vi "Runtime Test.vi"() -> ()   [LabVIEW 2017, in "WaveformAcq tests.lvlib"]
uses:
  WaveformAcq tests.lvlib
  <vilib>/NI/Tag Bus Module Framework/channel/channel classification.ctl
  <vilib>/NI/Tag Bus/tag/Data Type.ctl
  module/configuration/WaveformAcq configuration.lvclass
  C:/Program Files (x86)/National Instruments/LabVIEW 2017/vi.lib/NI/Configuration Framework/serializable configuration/NISE_CEF_serializable configuration.lvclass
  C:/Program Files (x86)/National Instruments/LabVIEW 2017/vi.lib/NI/Tag Bus Module Framework/module configuration/TBM module configuration.lvclass
  module/execution/WaveformAcq runtime.lvclass
  <vilib>/NI/Tag Bus/dictionary/data dictionary.lvclass/data dictionary.ctl
  <vilib>/NI/Tag Bus/dictionary/lookup polymorphs/locate double.vi
  <vilib>/NI/Tag Bus/table/data polymorphs/write one/write Double.vi
  <vilib>/NI/Tag Bus/table/data polymorphs/read one/read Double.vi
  <vilib>/NI/Tag Bus/dictionary/search/find data index.vi
  <vilib>/NI/Tag Bus/dictionary/search/search string list.vi
  <vilib>/NI/Tag Bus/dictionary/tag not found.vi
  <vilib>/NI/Tag Bus Module Framework/channel/TBM channel.lvclass
  <vilib>/NI/Tag Bus/tag/tag descriptor.lvclass
  <vilib>/NI/Tag Bus/dictionary/data dictionary.lvclass
  <vilib>/NI/Tag Bus/table/data table.lvlib
  <vilib>/NI/Configuration Framework/serializable configuration/NISE_CEF_serializable configuration.lvclass
panel:
  out "final error":errorcluster
  out "output error":errorcluster
  out "input error":errorcluster
  out "output lookup error":errorcluster
  out "no data written":bool
  out "input lookup error":errorcluster
  out "init error":errorcluster
  out "correct execution settings":bool
  out "serialization problem":errorcluster
  out "invalid configuration":errorcluster
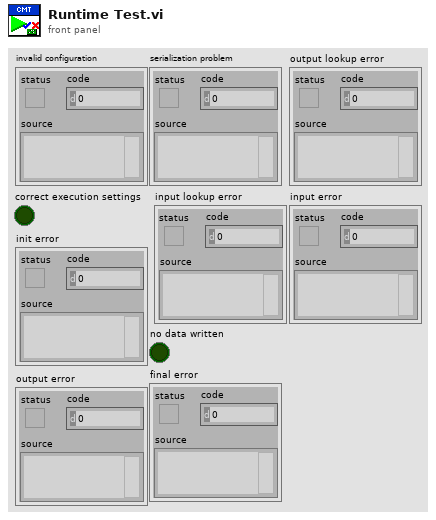
[diagram p1: front panel]
types:
  T1 = typedef "TBM channel.lvclass/channel classification.ctl" = enum16{"input data", "output data", "processing parameter", "processing result"}
  T2 = typedef "tag bus.lvlib/tag descriptor.lvclass/Data Type.ctl" = enum16{"Double", "Single", "I64", "I32", "I16", "I8", "U64", "U32", "U16", "U8", "Boolean", "String", "Array of Double", "Array of Single", "Array of I64", "Array of I32", "Array of I16", "Array of I8", "Array of U64", "Array of U32", "Array of U16", "Array of U8", "Array of Boolean", "Array of String"}
  T3 = cluster{"channel":refnum<class "TBM channel.lvclass">}
  T4 = typedef "TBM channel.lvclass/data tables.ctl" = cluster{"input data":T5, "processing parameter":T5, "processing result":T5, "output data":T5}
  T5 = typedef "tag bus.lvlib/dictionary table pair.ctl" = cluster{"data dictionary":refnum<class "data dictionary.lvclass">, "data table":T6}
  T6 = typedef "tag bus.lvlib/data table.lvlib/data table.ctl" = cluster{"Double":dbl[], "Single":sgl[], "I64":i64[], "I32":i32[], "I16":i16[], "I8":i8[], "U64":u64[], "U32":u32[], "U16":u16[], "U8":u8[], "Boolean":bool[], "String":string[], "Array of Double":cluster{"DBL Array":dbl[]}[], "Array of Single":cluster{"SGL Array":sgl[]}[], "Array of I64":cluster{"I64 Array":i64[]}[], "Array of I32":cluster{"I32 Array":i32[]}[], "Array of I16":cluster{"I16 Array":i16[]}[], "Array of I8":cluster{"I8 Array":i8[]}[], "Array of U64":cluster{"U64 Array":u64[]}[], "Array of U32":cluster{"U32 Array":u32[]}[], "Array of U16":cluster{"U16 Array":u16[]}[], "Array of U8":cluster{"U8 Array":u8[]}[], "Array of Boolean":cluster{"Boolean Array":bool[]}[], "Array of String":cluster{"String Array":string[]}[]}
  T7 = typedef "TBM module execution interface.lvclass/execution settings.ctl" = cluster{"reads inputs":bool, "processes data":bool, "writes outputs":bool}
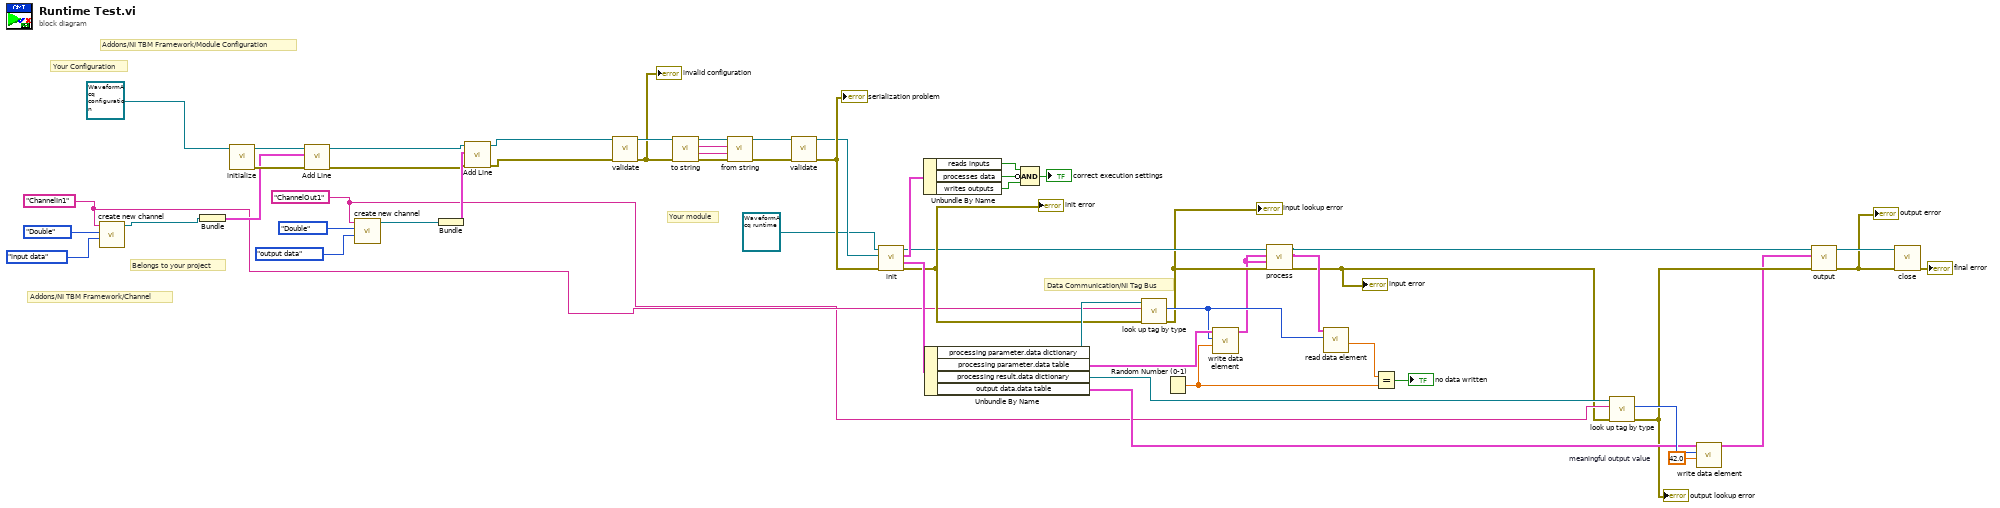
[diagram p0: block diagram]
diagram:
  w26 = 42.0  # meaningful output value
  w7 = "ChannelOut1" ("channel name")
  w8 = "ChannelIn1" ("channel name")
  # "Data Communication/NI Tag Bus"
  # "Your module"
  # "Your Configuration"
  # "Addons/NI TBM Framework/Module Configuration"
  # "Belongs to your project"
  # "Addons/NI TBM Framework/Channel"
  n1 = call <vilib>:"create new channel.vi"("channel classification"=channel_classification."input data", "data type"=Data_Type."Double", "channel name"=w8) -> ("channel"=w20:refnum<class "TBM channel.lvclass">)  [unwired: 8 in]
  n2 = Bundle("channel"=w20) -> (w10:T3)  [unwired: 1 in]
  n3 = call <vilib>:"initialize.vi"("configuration in"=refnum<class "WaveformAcq configuration.lvclass"> refnum ("user control module configuration")) -> ("error out"=w16:errorcluster, "configuration out"=w17:refnum<class "WaveformAcq configuration.lvclass">)  [unwired: 8 in, 1 out]
  n4 = call-dynamic "Add Line.vi"("error in (no error)"=w16, "Line"=w10, "WaveformAcq configuration in"=w17) -> ("error out"=w13:errorcluster, "WaveformAcq configuration out"=w15:refnum<class "WaveformAcq configuration.lvclass">)  [unwired: 7 in]
  n5 = call <vilib>:"create new channel.vi"("channel classification"=channel_classification."output data", "data type"=Data_Type."Double", "channel name"=w7) -> ("channel"=w19:refnum<class "TBM channel.lvclass">)  [unwired: 8 in]
  n6 = Bundle("channel"=w19) -> (w14:T3)  [unwired: 1 in]
  n7 = call-dynamic "Add Line.vi"("error in (no error)"=w13, "Line"=w14, "WaveformAcq configuration in"=w15) -> ("error out"=w12:errorcluster, "WaveformAcq configuration out"=w11:refnum<class "WaveformAcq configuration.lvclass">)  [unwired: 7 in]
  n8 = call-dynamic "validate.vi"("error in"=w12, "fixed channel configuration in"=w11) -> ("error out"=w51:errorcluster, "fixed channel configuration out"=w52:refnum<class "WaveformAcq configuration.lvclass">)  [unwired: 8 in]
  "invalid configuration" <- w51
  n9 = call-dynamic "to string.vi"("error in"=w51, "fixed channel configuration in"=w52) -> ("error out"=w47:errorcluster, "data"=w48:string, "version"=w49:string, "fixed channel configuration out"=w50:refnum<class "WaveformAcq configuration.lvclass">)  [unwired: 6 in]
  n10 = call-dynamic "from string.vi"("error in"=w47, "data"=w48, "version"=w49, "fixed channel configuration in"=w50) -> ("error out"=w45:errorcluster, "fixed channel configuration out"=w46:refnum<class "WaveformAcq configuration.lvclass">)  [unwired: 6 in]
  n11 = call-dynamic "validate.vi"("error in"=w45, "fixed channel configuration in"=w46) -> ("error out"=w44:errorcluster, "fixed channel configuration out"=w43:refnum<class "WaveformAcq configuration.lvclass">)  [unwired: 8 in]
  "serialization problem" <- w44
  n12 = call-dynamic "init.vi"("error in"=w44, "TBM module configuration in"=w43, "fixed channel runtime in"=refnum<class "WaveformAcq runtime.lvclass"> refnum ("user module")) -> ("error out"=w35:errorcluster, "data allocations"=w37:T4, "execution settings"=w42:T7, "fixed channel runtime out"=w6:refnum<class "WaveformAcq runtime.lvclass">)  [unwired: 5 in]
  "init error" <- w35
  n13 = Unbundle By Name(w42) -> ("reads inputs"=w39:bool, "processes data"=w41:bool, "writes outputs"=w40:bool)
  n14 = Unbundle By Name(w37) -> ("processing parameter.data dictionary"=w36:refnum<class "data dictionary.lvclass">, "processing parameter.data table"=w34:T6, "processing result.data dictionary"=w29:refnum<class "data dictionary.lvclass">, "output data.data table"=w27:T6)
  n15 = Compound Arithmetic op=AND(w39, invert w41, w40) -> (→"correct execution settings":bool)
  n16 = call-poly <vilib>:"look up tag by type.vi"("error in"=w35, "name"=w8, "data dictionary in"=w36) -> ("error out"=w3:errorcluster, "index"=w33:i32)  [unwired: 6 in, 1 out]
  "input lookup error" <- w3
  n17 = Random Number (0-1)() -> (number: 0 to 1=w32:dbl)
  n18 = call-poly <vilib>:"write data element.vi"("value"=w32, "index"=w33, "data table in"=w34) -> ("data table out"=w1:T6)  [unwired: 8 in]
  n19 = call-dynamic "process.vi"("error in"=w3, "result allocation"=w1, "parameters"=w1, "WaveformAcq runtime in"=w6) -> ("error out"=w2:errorcluster, "parameter allocation"=w4:T6, "WaveformAcq runtime out"=w5:refnum<class "WaveformAcq runtime.lvclass">)  [unwired: 4 in, 1 out]
  "input error" <- w2
  n20 = call-poly <vilib>:"read data element.vi"("index"=w33, "data table in"=w4) -> ("value"=w31:dbl)  [unwired: 8 in, 1 out]
  n21 = Equal?(x=w31, y=w32) -> (x = y?=→"no data written":bool)
  n22 = call-poly <vilib>:"look up tag by type.vi"("error in"=w2, "name"=w7, "data dictionary in"=w29) -> ("error out"=w25:errorcluster, "index"=w28:i32)  [unwired: 6 in, 1 out]
  "output lookup error" <- w25
  n23 = call-poly <vilib>:"write data element.vi"("value"=w26, "index"=w28, "data table in"=w27) -> ("data table out"=w24:T6)  [unwired: 8 in]
  n24 = call-dynamic "output.vi"("error in"=w25, "output data"=w24, "WaveformAcq runtime in"=w5) -> ("error out"=w22:errorcluster, "WaveformAcq runtime out"=w23:refnum<class "WaveformAcq runtime.lvclass">)  [unwired: 6 in, 1 out]
  "output error" <- w22
  n25 = call-dynamic "close.vi"("error in"=w22, "module in"=w23) -> ("error out"=→"final error":errorcluster)  [unwired: 9 in]
